vi "initialize_camera_settings.vi"(3 "Trigger":u32(ring) items=["Internal", "External"], 4 "Exposure \ntime (secs)":dbl=0.005 format="%.3f") -> ()   [LabVIEW 2011]
uses:
  <userlib>/atmcd32d.llb/Shutter_type typedef.ctl
panel:
  # "Camera settings"
  # "Frame rate (ms)"
  # "Status"
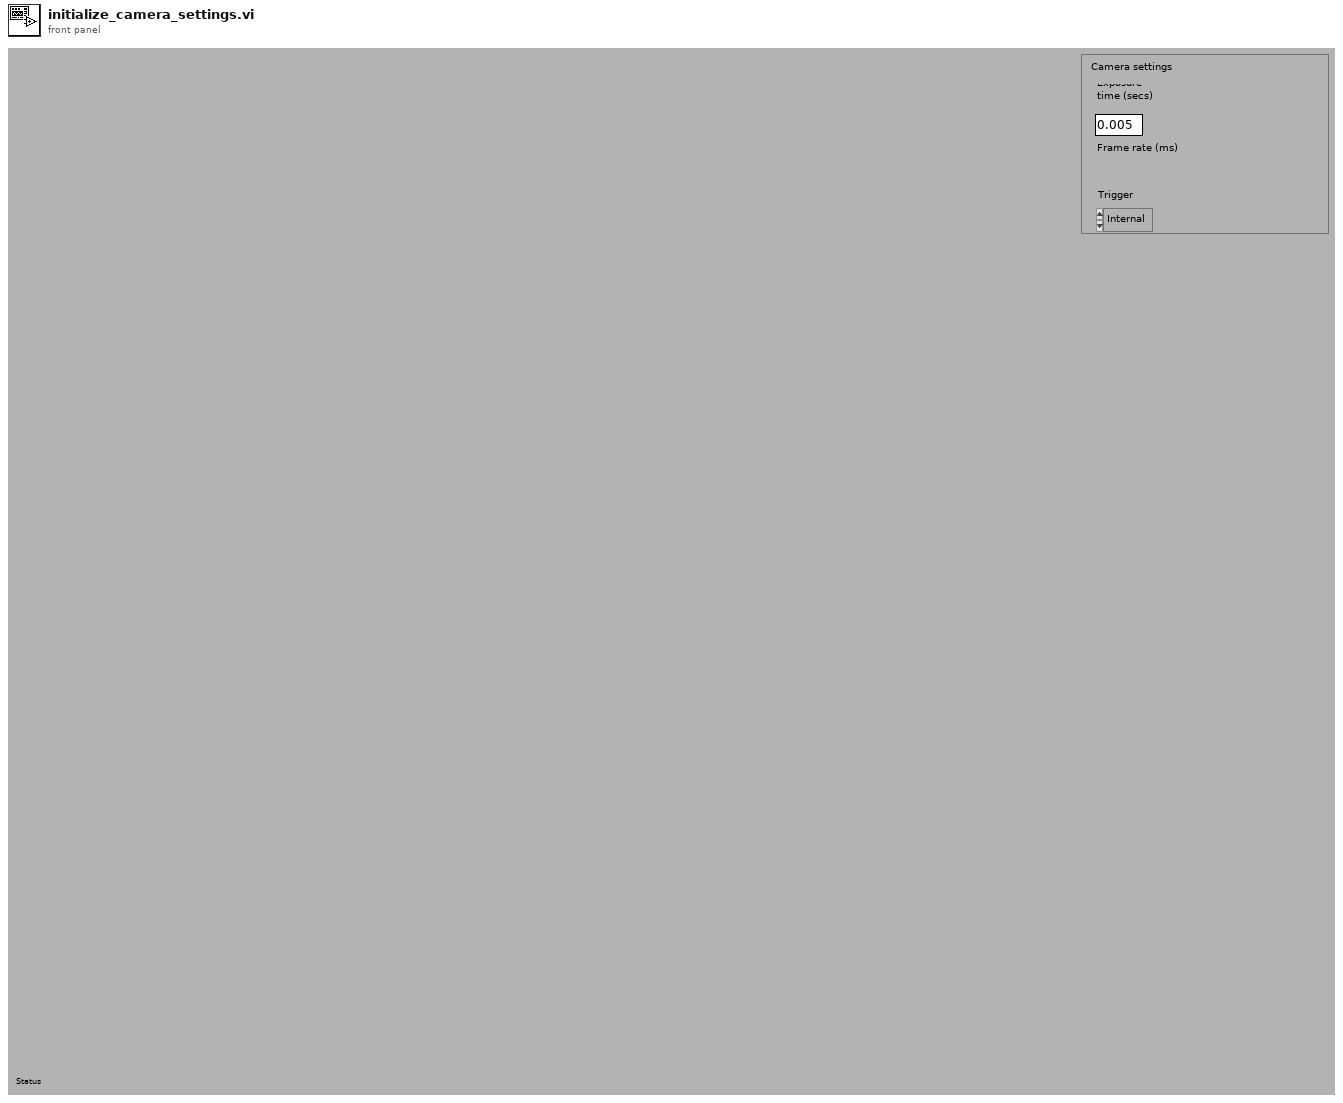
[diagram p1: front panel]
types:
  T1 = typedef "Shutter_type typedef.ctl" = enum16{"TTL Low", "TTL High"}
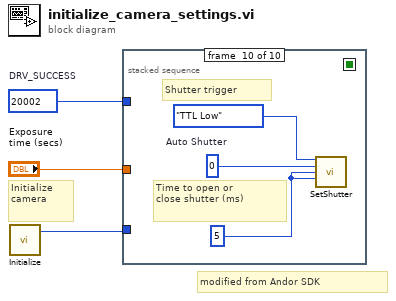
[diagram p0: block diagram]
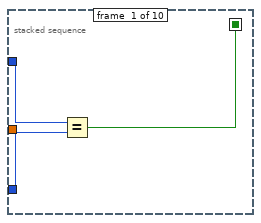
[diagram p2: hidden frame]
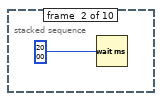
[diagram p3: hidden frame]
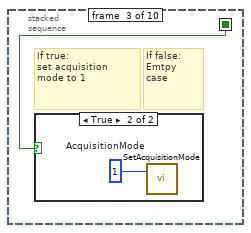
[diagram p4: hidden frame]
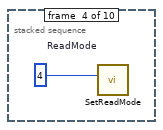
[diagram p6: hidden frame]
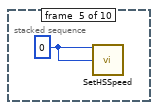
[diagram p7: hidden frame]
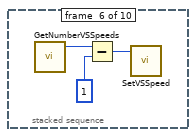
[diagram p8: hidden frame]
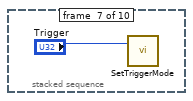
[diagram p9: hidden frame]
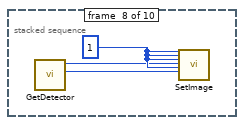
[diagram p10: hidden frame]
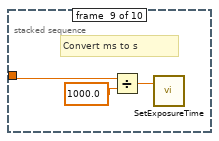
[diagram p11: hidden frame]
diagram:
  w2 = 20002  # DRV_SUCCESS
  # "Initialize\ncamera"
  # "modified from Andor SDK"
  n1 = call <userlib>:"Initialize.vi"() -> ("DLL error code"=w3:u32)  [unwired: 2 in, 1 out]
  n2 = stacked-sequence {
    seq-local: [w4 _ _ _ _ _ _ _ _ _] -> [_ _ w8 _ _ _ _ _ _ _]
    tunnel: "Exposure \ntime (secs)" -> [_ _ _ _ _ _ _ _ w21 _]
    tunnel: w2 -> [w6 _ _ _ _ _ _ _ _ _]
    tunnel: w3 -> [w5 _ _ _ _ _ _ _ _ _]
    frame #0 {
      n3 = Equal?(x=w6, y=w5) -> (x = y?=w4:bool)
    }
    frame #1 {
      n4 = Wait (ms)(milliseconds to wait=u32 2000) -> ()  [unwired: 1 out]
    }
    frame #2 {
      # "If false:\nEmtpy\ncase"
      # "If true:\nset acquisition\nmode to 1"
      n5 = case shown="True" w8 {
        frame False {
        }
        frame True {
          w9 = u16 1  # AcquisitionMode
          n6 = call <userlib>:"SetAcquisitionMode.vi"("mode"=w9) -> ()  [unwired: 1 in, 2 out]
        }
      }
    }
    frame #3 {
      w10 = u16 4  # ReadMode
      n7 = call <userlib>:"SetReadMode.vi"("mode"=w10) -> ()  [unwired: 1 in, 2 out]
    }
    frame #4 {
      w11 = 0
      n8 = call <userlib>:"SetHSSpeed.vi"("index"=w11, "type"=w11) -> ()  [unwired: 2 in, 2 out]
    }
    frame #5 {
      n9 = call <userlib>:"GetNumberVSSpeeds.vi"() -> ("number"=w14:i32)  [unwired: 3 in, 2 out]
      n10 = Subtract(x=w14, y=1) -> (x-y=w12:i32)
      n11 = call <userlib>:"SetVSSpeed.vi"("index"=w12) -> ()  [unwired: 1 in, 2 out]
    }
    frame #6 {
      n12 = call <userlib>:"SetTriggerMode.vi"("mode"="Trigger") -> ()  [unwired: 1 in, 2 out]
    }
    frame #7 {
      w18 = 1 ("hbin")
      n13 = call <userlib>:"GetDetector.vi"() -> ("ypixels"=w16:i32, "xpixels"=w17:i32)  [unwired: 4 in, 2 out]
      n14 = call <userlib>:"SetImage.vi"("hbin"=w18, "vbin"=w18, "hstart"=w18, "hend"=w17, "vstart"=w18, "vend"=w16) -> ()  [unwired: 20 in, 2 out]
    }
    frame #8 {
      # "Convert ms to s"
      n15 = Divide(x=w21, y=1000.0) -> (x/y=w19:dbl)
      n16 = call <userlib>:"SetExposureTime.vi"("time"=w19) -> ()  [unwired: 1 in, 2 out]
    }
    frame #9 {
      w23 = 5 ("closingtime")
      w24 = 0  # Auto Shutter
      # "Shutter trigger"
      # "Time to open or\nclose shutter (ms)"
      n17 = call <userlib>:"SetShutter.vi"("type"=Shutter_type_typedef."TTL Low", "mode"=w24, "closingtime"=w23, "openingtime"=w23) -> ()  [unwired: 10 in, 2 out]
    }
  }
